vi "ABAPI Dist append to array if not present.vi"(2 "new elements":u32[](array[numeric]), 3 "array in":u32[](array[numeric])) -> (1 "array out":u32[](array[numeric]))   [LabVIEW 2020]
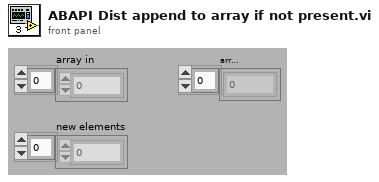
[diagram p1: front panel]
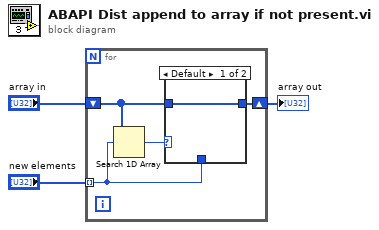
[diagram p0: block diagram]
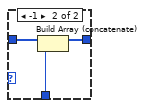
[diagram p2: hidden frame]
diagram:
  n1 = for {
    shift-right: [w6] -> w2
    shift-left: "array in" -> [w4]
    tunnel: "new elements" -> [w5] mode=indexing
    n2 = Search 1D Array(1D array=w4, element=w5) -> (index of element=w7:i32)  [unwired: 1 in]
    n3 = case shown="Default" w7 {
      tunnel: [w8 w10] -> w6
      tunnel: w4 -> [w8 w11]
      tunnel: w5 -> [_ w9]
      frame Default {
      }
      frame -1 {
        n4 = Build Array (concatenate)(w11, w9) -> (w10:u32[])
      }
    }
  }
  "array out" <- w2
